vi "Receive Event.vi"(8 "Error In":errorcluster, 9 "Event Data":refnum<class "Event Data.lvclass">, 10 "Event Name":string, 11 "Server In":refnum<class "Server.lvclass">) -> (0 "Error Out":errorcluster, 3 "Server Out":refnum<class "Server.lvclass">)   [LabVIEW 2020, in "Server.lvlib" / "Server.lvclass"]
uses:
  Server.lvclass
  C:/Program Files/National Instruments/LabVIEW 2020/vi.lib/ActorFramework/Actor/Actor.lvclass
  SubPanel-Actor-Framework-master/Event-Source-Actor/Source/Template Source/Event Data/Event Data.lvclass
  <vilib>/ActorFramework/Actor/Actor.lvclass/Actor.ctl
  <vilib>/ActorFramework/Message Enqueuer/Message Enqueuer.lvclass/Message Enqueuer.ctl
  Event-Source-Actor/Data Interface/Message Data/Message Data.lvclass
  Server Messages/Direct Message Recieved Msg/Direct Message Recieved Msg.lvclass/Direct Message Recieved Msg.ctl
  Event-Source-Actor/Data Interface/VI Info Data/VI Info Data.lvclass
  Server Messages/New Reference Recieved Msg/New Reference Recieved Msg.lvclass/New Reference Recieved Msg.ctl
  Event-Source-Actor/Data Interface/Status Data/Status Data.lvclass
  <vilib>/ActorFramework/Message Enqueuer/Init from Existing Queue.vi
  <vilib>/ActorFramework/Message Enqueuer/Enqueue.vi
  Server Messages/Direct Message Recieved Msg/Direct Message Recieved Msg.lvclass
  C:/Program Files/National Instruments/LabVIEW 2020/vi.lib/ActorFramework/Message/Message.lvclass
  Server Messages/New Reference Recieved Msg/New Reference Recieved Msg.lvclass
  <vilib>/ActorFramework/Message Priority Queue/Priority Enqueue.vi
  <vilib>/ActorFramework/Message Enqueuer/Message Enqueuer.lvclass
  <vilib>/ActorFramework/Actor/Actor.lvclass
  Server Messages/Status Update Msg/Status Update Msg.lvclass
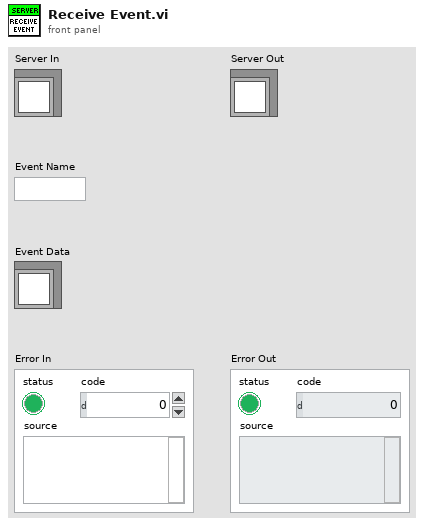
[diagram p1: front panel]
types:
  T1 = typedef "Message Control.ctl" = cluster{"From":string, "To":string, "Message":string}
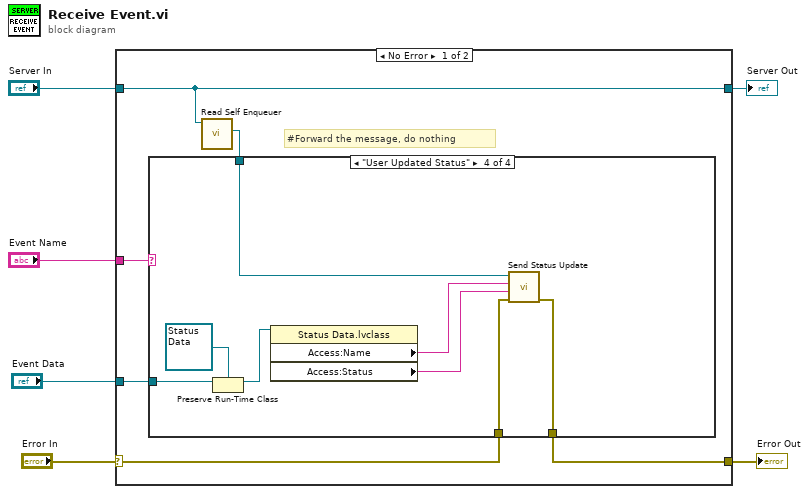
[diagram p0: block diagram]
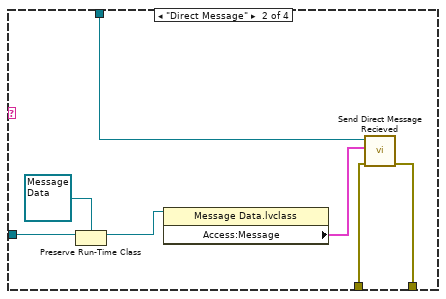
[diagram p3: hidden frame]
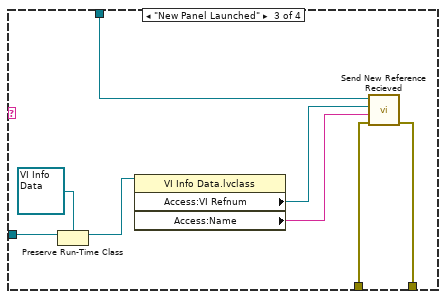
[diagram p4: hidden frame]
diagram:
  n1 = case shown="No Error" "Error In" {
    selector: "Error In" -> [w10 w37]
    tunnel: [w8 w38] -> w6
    tunnel: "Server In" -> [w8 w38]
    tunnel: [w9 w37] -> w3
    tunnel: "Event Name" -> [w12 _]
    tunnel: "Event Data" -> [w11 _]
    frame No Error {
      # "#Forward the message, do nothing"
      n2 = call <vilib>:"Read Self Enqueuer.vi"("Actor"=w8) -> ("Self Enqueuer"=w7:refnum<class "Message Enqueuer.lvclass">)  [unwired: 10 in]
      n3 = case shown="\"User Updated Status\"" w12 {
        tunnel: w11 -> [_ w19 w27 w35]
        tunnel: w10 -> [w13 w16 w22 w30]
        tunnel: [w13 w14 w21 w29] -> w9
        tunnel: w7 -> [_ w17 w25 w33]
        frame "False", Default {
        }
        frame "Direct Message" {
          n4 = Preserve Run-Time Class(object in=w19, 2:refnum<class "Message Data.lvclass"> refnum ("Message Data.lvclass")) -> (object out=w18:refnum<class "Message Data.lvclass">)  [unwired: 1 in, 1 out]
          n5 = property class="Message Data.lvclass"(reference=w18) -> ("Access:Message"=w15:T1)  [unwired: 1 in, 2 out]
          n6 = call "Send Direct Message Recieved.vi"("error in (no error)"=w16, "Message"=w15, "Message Enqueuer in"=w17) -> ("error out"=w14:errorcluster)  [unwired: 7 in, 1 out]
        }
        frame "New Panel Launched" {
          n7 = Preserve Run-Time Class(object in=w27, 2:refnum<class "VI Info Data.lvclass"> refnum ("VI Info Data.lvclass")) -> (object out=w26:refnum<class "VI Info Data.lvclass">)  [unwired: 1 in, 1 out]
          n8 = property class="VI Info Data.lvclass"(reference=w26) -> ("Access:VI Refnum"=w24:refnum<vi>, "Access:Name"=w23:string)  [unwired: 1 in, 2 out]
          n9 = call "Send New Reference Recieved.vi"("error in (no error)"=w22, "Name"=w23, "VI Refnum"=w24, "Message Enqueuer in"=w25) -> ("error out"=w21:errorcluster)  [unwired: 6 in, 1 out]
        }
        frame "User Updated Status" {
          n10 = Preserve Run-Time Class(object in=w35, 2:refnum<class "Status Data.lvclass"> refnum ("Status Data.lvclass")) -> (object out=w34:refnum<class "Status Data.lvclass">)  [unwired: 1 in, 1 out]
          n11 = property class="Status Data.lvclass"(reference=w34) -> ("Access:Name"=w32:string, "Access:Status"=w31:string)  [unwired: 1 in, 2 out]
          n12 = call "Send Status Update.vi"("error in (no error)"=w30, "Status"=w31, "Name"=w32, "Message Enqueuer in"=w33) -> ("error out"=w29:errorcluster)  [unwired: 6 in, 1 out]
        }
      }
    }
    frame Error {
    }
  }
  "Server Out" <- w6
  "Error Out" <- w3
